vi "Get Reader Timestamp.vi"(10 "ID":string="Reader", 11 "data attributes":variant) -> (1 "timestamp":timestamp format="%<%H:%M:%S%6u\n%x>T", 3 "data attributes":variant)   [LabVIEW 2017]
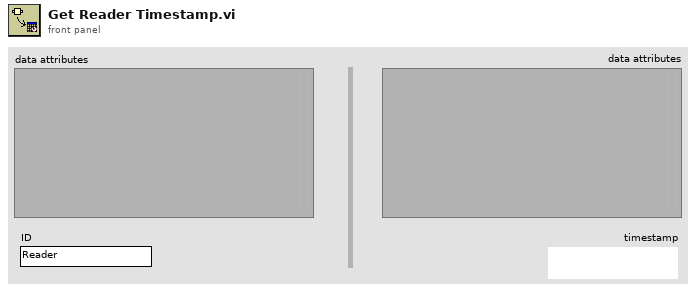
[diagram p1: front panel]
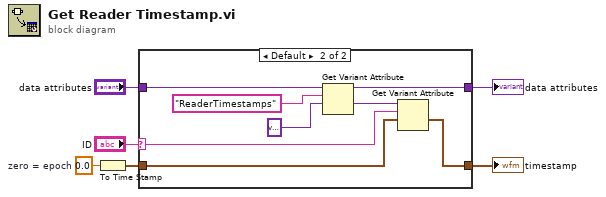
[diagram p0: block diagram]
diagram:
  w2 = 0.0  # zero = epoch
  n1 = To Time Stamp(1:w2) -> (0:w1:timestamp)
  n2 = case shown="Default" "ID" {
    selector: "ID" -> [_ w10]
    tunnel: [w7 w16] -> w6
    tunnel: [w8 w13] -> w5
    tunnel: "data attributes" -> [w8 w12]
    tunnel: w1 -> [w7 w9]
    frame "" {
    }
    frame Default {
      n3 = Get Variant Attribute(Variant=w12, name="ReaderTimestamps", default value (empty Variant)=variant ("ReaderTimestamps")) -> (duplicate Variant=w13:variant, value=w11:variant)  [unwired: 1 in, 2 out]
      n4 = Get Variant Attribute(Variant=w11, name=w10, default value (empty Variant)=w9) -> (value=w16:timestamp)  [unwired: 1 in, 3 out]
    }
  }
  "data attributes" <- w5
  "timestamp" <- w6
